vi "BuildRelease_AddStatesToQueue.vi"(0 "State(s) in Front (\"\")":string, 2 "EmptyQueueNextState":string, 5 "State(s) in (\"\")":string, 7 "State(s) at Back (\"\")":string) -> (6 "States Out":string)   [LabVIEW 2016]
doc: "<B>Inputs:</B>\n <B>State(s) in Front:</B> This allows you to place new states in the front of the state machine queue. The default is an empty string.\n <B>State(s) in:</B> Wire the existing states to this input. The default is an empty string.\n <B>State(s) in Back:</B> This allows you to place new states in the back of the state machine queue. The default is an empty string.\n <B>EmptyQueueNextState</B> This state will only be used if there are no other states to process. The default is an empty string.\n\n<B>Outputs:</B>\n <B>States Out:</B>This output returns a concatenation of all the inputs seperated by a line feed character."
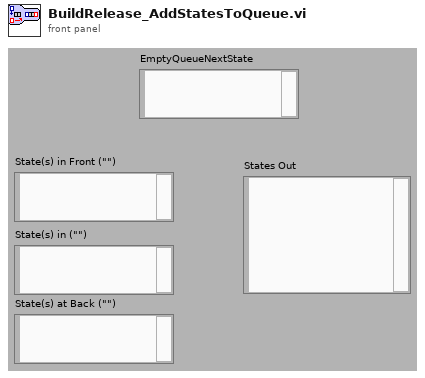
[diagram p1: front panel]
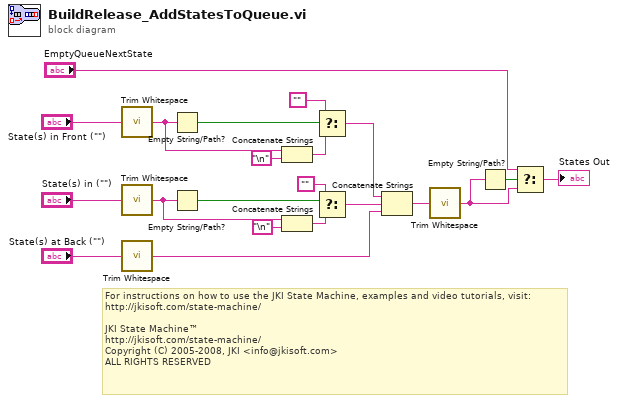
[diagram p0: block diagram]
diagram:
  # "For instructions on how to use the JKI State Machine, examples and video tutorials, visit:\nhttp://jkisoft.com/state-machine/\n\nJKI State Machine™\nhttp://jkisoft.com/state-machine/\nCopyright (C) 2005-2008, JKI <info@jkisoft.com>\nALL RIGHTS RESERVED"
  n1 = call <vilib>:"Trim Whitespace.vi"("string"="State(s) in Front (\"\")") -> ("trimmed string"=w14:string)  [unwired: 1 in]
  n2 = call <vilib>:"Trim Whitespace.vi"("string"="State(s) in (\"\")") -> ("trimmed string"=w10:string)  [unwired: 1 in]
  n3 = call <vilib>:"Trim Whitespace.vi"("string"="State(s) at Back (\"\")") -> ("trimmed string"=w9:string)  [unwired: 1 in]
  n4 = Empty String/Path?(string/path=w14) -> (empty?=w18:bool)
  n5 = Empty String/Path?(string/path=w10) -> (empty?=w8:bool)
  n6 = Concatenate Strings(w14, "\n") -> (w13:string)
  n7 = Concatenate Strings(w10, "\n") -> (w11:string)
  n8 = Select(t="", s=w18, f=w13) -> (s? t:f=w17:string)
  n9 = Select(t="", s=w8, f=w11) -> (s? t:f=w16:string)
  n10 = Concatenate Strings(w17, w16, w9) -> (w5:string)
  n11 = call <vilib>:"Trim Whitespace.vi"("string"=w5) -> ("trimmed string"=w2:string)  [unwired: 1 in]
  n12 = Empty String/Path?(string/path=w2) -> (empty?=w4:bool)
  n13 = Select(t="EmptyQueueNextState", s=w4, f=w2) -> (s? t:f=→"States Out":string)
